vi "decoder 3 to 8.vi"() -> ()   [LabVIEW 2020]
panel:
  out "A7":bool
  out "A6":bool
  out "A5":bool
  out "A4":bool
  out "A3":bool
  out "A2":bool
  out "A1":bool
  out "A0":bool
  in  "Boolean 3":bool
  in  "Boolean 2":bool
  in  "Boolean":bool
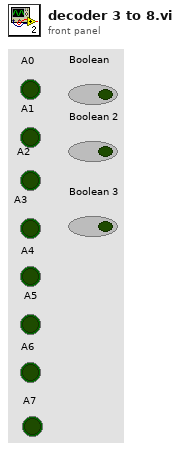
[diagram p1: front panel]
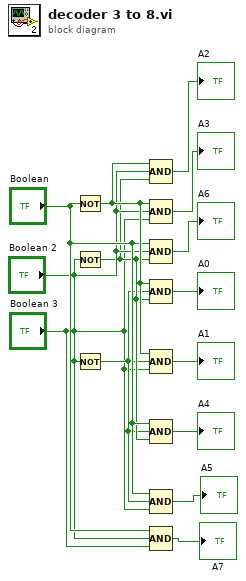
[diagram p0: block diagram]
diagram:
  n1 = Not(x="Boolean") -> (.not. x?=w14:bool)
  n2 = Not(x="Boolean 3") -> (.not. x?=w11:bool)
  n3 = Not(x="Boolean 2") -> (.not. x?=w10:bool)
  n4 = Compound Arithmetic op=AND(w14, "Boolean 2", w11) -> (→"A2":bool)
  n5 = Compound Arithmetic op=AND(w14, "Boolean 2", "Boolean 3") -> (→"A3":bool)
  n6 = Compound Arithmetic op=AND("Boolean", "Boolean 2", w11) -> (→"A6":bool)
  n7 = Compound Arithmetic op=AND(w14, w10, w11) -> (→"A0":bool)
  n8 = Compound Arithmetic op=AND(w14, w10, "Boolean 3") -> (→"A1":bool)
  n9 = Compound Arithmetic op=AND("Boolean", w10, w11) -> (→"A4":bool)
  n10 = Compound Arithmetic op=AND("Boolean", w10, "Boolean 3") -> (→"A5":bool)
  n11 = Compound Arithmetic op=AND("Boolean", "Boolean 2", "Boolean 3") -> (→"A7":bool)
